vi "Initialize_Images_Array_Random_Names-1.vi"(1 "error IN":errorcluster, 2 "# Pics":i32, 3 "Image Type":T1 items=["Grayscale (U8)", "Grayscale (I16)", "Grayscale (SGL)", "Complex (CSG)", "RGB (U32)", "HSL (U32)", "RGB (U64)", "Grayscale (U16)"]) -> (0 "Images Array":T2[](array[typedef]))   [LabVIEW 2013]
uses:
  <vilib>/vision/Image Controls.llb/IMAQ Image.ctl
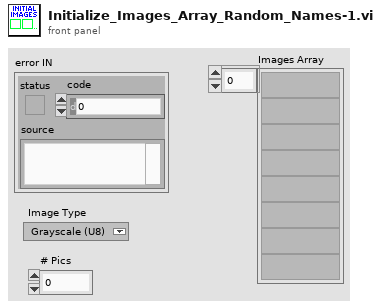
[diagram p1: front panel]
types:
  T1 = typedef "Image Type" = u32
  T2 = typedef "IMAQ Image.ctl" = refnum<image>
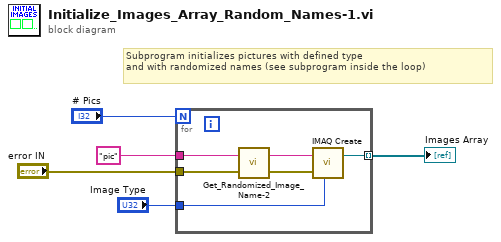
[diagram p0: block diagram]
diagram:
  # "Subprogram initializes pictures with defined type \nand with randomized names (see subprogram inside the loop)"
  n1 = for {
    N: "# Pics" -> [_]
    tunnel: "error IN" -> [w8]
    tunnel: [w11] -> w3 mode=indexing
    tunnel: "Image Type" -> [w10]
    tunnel: "pic" ("Main Name") -> [w9]
    n2 = call "Get_Randomized_Image_Name-2.vi"("error IN"=w8, "Main Name"=w9) -> ("error OUT"=w6:errorcluster, "Randomized name"=w7:string)
    n3 = call "IMAQ Create"("Image Name"=w7, "Image Type"=w10, "error in (no error)"=w6) -> ("New Image"=w11:T2)  [unwired: 2 in, 1 out]
  }
  "Images Array" <- w3
